vi "MGI Error Queue Flush.vi"(8 "error in (no error)":errorcluster, 11 "MGI Error Reporter Base In":refnum<class "MGI Error Reporter Base.lvclass">) -> (0 "error out":errorcluster, 2 "Error[]":errorcluster[](array[cluster]))   [LabVIEW 2016, in "MGI Error Reporter Base.lvclass"]
doc: "Output True if the Error Queue is valid.\nThis VI behaves differently on different targets.\n\nAuthored by Shawn Walpole\nsupport@mooregoodideas.com\nwww.mooregoodideas.com\n\nCopyright (c) 2013, Moore Good Ideas, Inc.\n\nAll rights reserved.\n\nRedistribution and use in source and binary forms, with or without modification, are permitted provided that the following conditions are met:\n\n * Redistributions of source code must retain the above copyright notice, this list of conditions and the following disclaimer.\n * Redistributions in binary form must reproduce the above copyright notice, this list of conditions and the following disclaimer in the documentation and/or other materials provided with the distribution.\n * Neither the name of Moore Good Ideas, Inc. nor the names of its contributors may be used to endorse or promote products derived from this software without specific prior written permission.\n\nTHIS SOFTWARE IS PROVIDED BY THE COPYRIGHT HOLDERS AND CONTRIBUTORS \"AS IS\" AND ANY EXPRESS OR IMPLIED WARRANTIES, INCLUDING, BUT NOT LIMITED TO, THE IMPLIED WARRANTIES OF MERCHANTABILITY AND FITNESS FOR A PARTICULAR PURPOSE ARE DISCLAIMED. IN NO EVENT SHALL THE COPYRIGHT OWNER OR CONTRIBUTORS BE LIABLE FOR ANY DIRECT, INDIRECT, INCIDENTAL, SPECIAL, EXEMPLARY, OR CONSEQUENTIAL DAMAGES (INCLUDING, BUT NOT LIMITED TO, PROCUREMENT OF SUBSTITUTE GOODS OR SERVICES; LOSS OF USE, DATA, OR PROFITS; OR BUSINESS INTERRUPTION) HOWEVER CAUSED AND ON ANY THEORY OF LIABILITY, WHETHER IN CONTRACT, STRICT LIABILITY, OR TORT (INCLUDING NEGLIGENCE OR OTHERWISE) ARISING IN ANY WAY OUT OF THE USE OF THIS SOFTWARE, EVEN IF ADVISED OF THE POSSIBILITY OF SUCH DAMAGE."
uses:
  <userlib>/_MGI/Error Reporter/MGI Error Reporter Base/MGI Error Reporter Base.lvclass
  <userlib>/_MGI/Error Reporter/MGI Error Reporter Base/MGI Error Reporter Base.lvclass/MGI Error Reporter Base.ctl
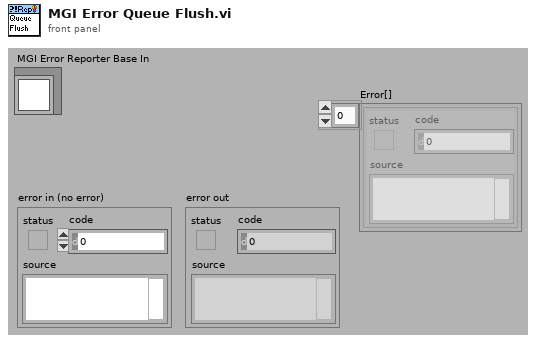
[diagram p1: front panel]
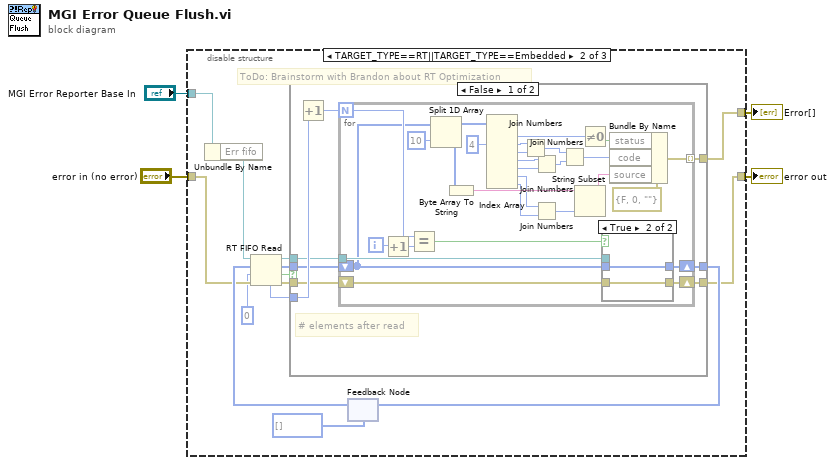
[diagram p0: block diagram]
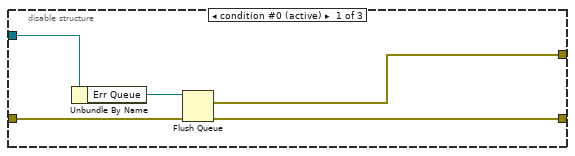
[diagram p2: hidden frame]
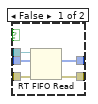
[diagram p3: hidden frame]
diagram:
  n1 = disable-structure shown="TARGET_TYPE==RT||TARGET_TYPE==Embedded" {
    disable-tunnel: [w9 w13 _] -> w4
    disable-tunnel: [w8 w12 _] -> w3
    disable-tunnel: "error in (no error)" -> [w7 w19 _]
    disable-tunnel: "MGI Error Reporter Base In" -> [w6 w11 _]
    frame condition #0 (active) {
      n2 = Unbundle By Name(w6) -> ("Err Queue"=w5:refnum<queue>)
      n3 = Flush Queue(queue=w5, error in (no error)=w7) -> (remaining elements=w9:errorcluster[], error out=w8:errorcluster)  [unwired: 1 out]
    }
    frame condition #1 {
      # "ToDo: Brainstorm with Brandon about RT Optimization"
      n4 = Unbundle By Name(w11) -> ("Err fifo"=w10:refnum<k33>)
      n5 = feedback #1(u8[] [] ("element out")) -> (w22:u8[])
      n6 = RT FIFO Read(0:w10, 1:w22, 2:0 ("timeout in ms (0)"), 3:w19) -> (7:w21:u32, 8:w20:refnum<k33>, 9:w17:u8[], 10:w15:bool, 11:w18:errorcluster)
      n7 = case shown="False" w15 {
        tunnel: w21 -> [w31 _]
        tunnel: w20 -> [w30 _]
        tunnel: w18 -> [w29 w69]
        tunnel: w17 -> [w28 w68]
        tunnel: [w24 w69] -> w12
        tunnel: [w26 w68] -> w14
        tunnel: [w25 _] -> w13
        frame False {
          # "# elements after read"
          n8 = Increment(x=w31) -> (x+1=w27:u32)
          n9 = for {
            N: w27 -> [w56]
            tunnel: w30 -> [w60]
            shift-right: [w57] -> w24
            shift-left: w29 -> [w58]
            shift-right: [w59] -> w26
            shift-left: w28 -> [w36]
            tunnel: [w35] -> w25 mode=indexing
            i -> [w55]
            n10 = Increment(x=w55) -> (x+1=w54:i32)
            n11 = Equal?(x=w56, y=w54) -> (x = y?=w53:bool)
            n12 = Split 1D Array(array=w36, index=10) -> (first subarray=w41:u8[], second subarray=w38:u8[])
            n13 = Byte Array To String(unsigned byte array=w38) -> (string=w40:string)
            n14 = Index Array(array=w41, index #2=4 ("index")) -> (element #1=w42:u8, element #2=w45:u8, element #3=w46:u8, element #4=w47:u8, element #5=w48:u8, element #6=w33:u8, element #7=w34:u8)  [unwired: 6 in]
            n15 = Join Numbers(hi=w45, lo=w46) -> ((hi.lo)=w49:u16)
            n16 = Join Numbers(hi=w47, lo=w48) -> ((hi.lo)=w50:u16)
            n17 = Join Numbers(hi=w33, lo=w34) -> ((hi.lo)=w32:u16)
            n18 = Join Numbers(hi=w49, lo=w50) -> ((hi.lo)=w51:u32)
            n19 = String Subset(string=w40, length (rest)=w32) -> (substring=w52:string)  [unwired: 1 in]
            n20 = Not Equal To 0?(x=w42) -> (x != 0?=w43:bool)
            n21 = case shown="True" w53 {
              tunnel: w60 -> [w65 _]
              tunnel: [w64 w66] -> w59
              tunnel: w58 -> [w63 w67]
              tunnel: [w62 w67] -> w57
              tunnel: w36 -> [w61 w66]
              frame False {
                n22 = RT FIFO Read(0:w65, 1:w61, 3:w63) -> (9:w64:u8[], 11:w62:errorcluster)  [unwired: 1 in, 3 out]
              }
              frame True {
              }
            }
            n23 = Bundle By Name(cluster=errorcluster {"status"=FALSE, "code"=0, "source"=""} ("error in (no error)"), "status"=w43, "code"=w51, "source"=w52) -> (w35:errorcluster)
          }
        }
        frame True {
        }
      }
      n24 = feedback-in #1(w14) -> ()
    }
    frame condition #2 {
      # "Not handled"
    }
  }
  "Error[]" <- w4
  "error out" <- w3
